vi "Blob Scoring.vi"(8 "HSL Image":T2, 11 "Acceptable Blobs":T4(array[cluster])) -> (3 "Acceptable Blobs + Scores":T3(array[cluster]))   [LabVIEW 2014]
uses:
  <vilib>/vision/Image Controls.llb/IMAQ Image.ctl
  <vilib>/vision/NI_Vision_Development_Module.lvlib
panel:
  in  "Particle Report":T1
  in  "Upper Limit Y":dbl[](array[numeric])
  in  "Lower Limit Y":dbl[](array[numeric])=[0.7, 0.7, 0.7, 0.7, 0.7, 0.7, 0.2, 0.2, 0.2, 0.2, 0.2, 0.2, 0.2, 0.2, 0.2, 0.2, 0.2, 0.2, 0.2, 0.2, 0.2]
  in  "Upper Limit X":dbl[](array[numeric])
  in  "Lower Limit X":dbl[](array[numeric])
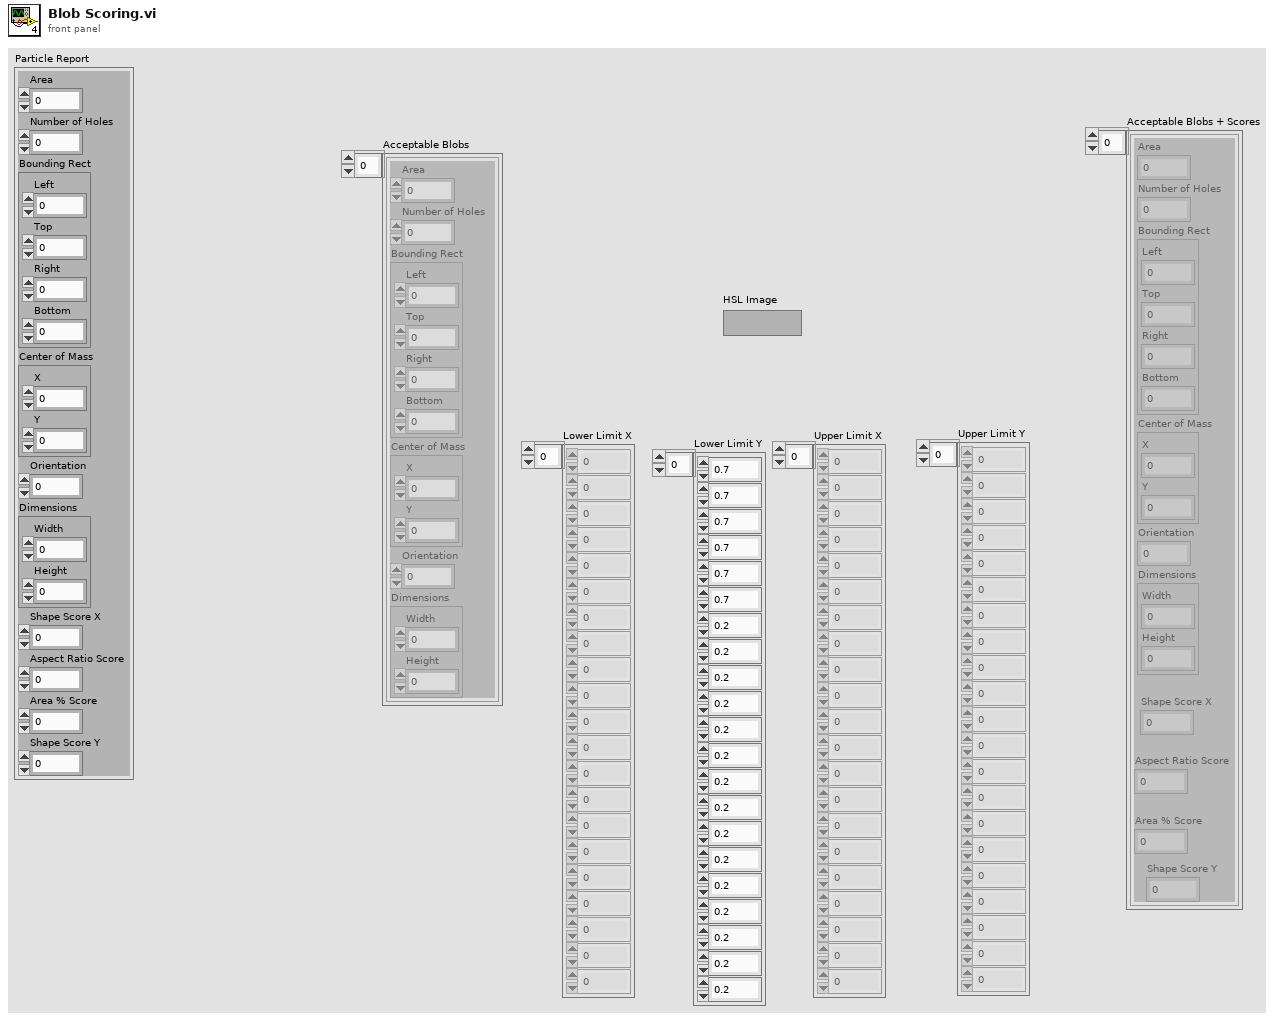
[diagram p1: front panel]
types:
  T1 = cluster{"Area":dbl, "Number of Holes":dbl, "Bounding Rect":cluster{"Left":dbl, "Top":dbl, "Right":dbl, "Bottom":dbl}, "Center of Mass":cluster{"X":dbl, "Y":dbl}, "Orientation":dbl, "Dimensions":cluster{"Width":dbl, "Height":dbl}, "Shape Score X":dbl, "Aspect Ratio Score":dbl, "Area % Score":dbl, "Shape Score Y":dbl}
  T2 = typedef "IMAQ Image.ctl" = refnum<image>
  T3 = cluster{"Area":dbl, "Number of Holes":dbl, "Bounding Rect":cluster{"Left":dbl, "Top":dbl, "Right":dbl, "Bottom":dbl}, "Center of Mass":cluster{"X":dbl, "Y":dbl}, "Orientation":dbl, "Dimensions":cluster{"Width":dbl, "Height":dbl}, "Shape Score X":dbl, "Aspect Ratio Score":dbl, "Area % Score":dbl, "Shape Score Y":dbl}[]
  T4 = cluster{"Area":dbl, "Number of Holes":dbl, "Bounding Rect":cluster{"Left":dbl, "Top":dbl, "Right":dbl, "Bottom":dbl}, "Center of Mass":cluster{"X":dbl, "Y":dbl}, "Orientation":dbl, "Dimensions":cluster{"Width":dbl, "Height":dbl}}[]
  T5 = cluster{"Left":dbl, "Top":dbl, "Right":dbl, "Bottom":dbl}
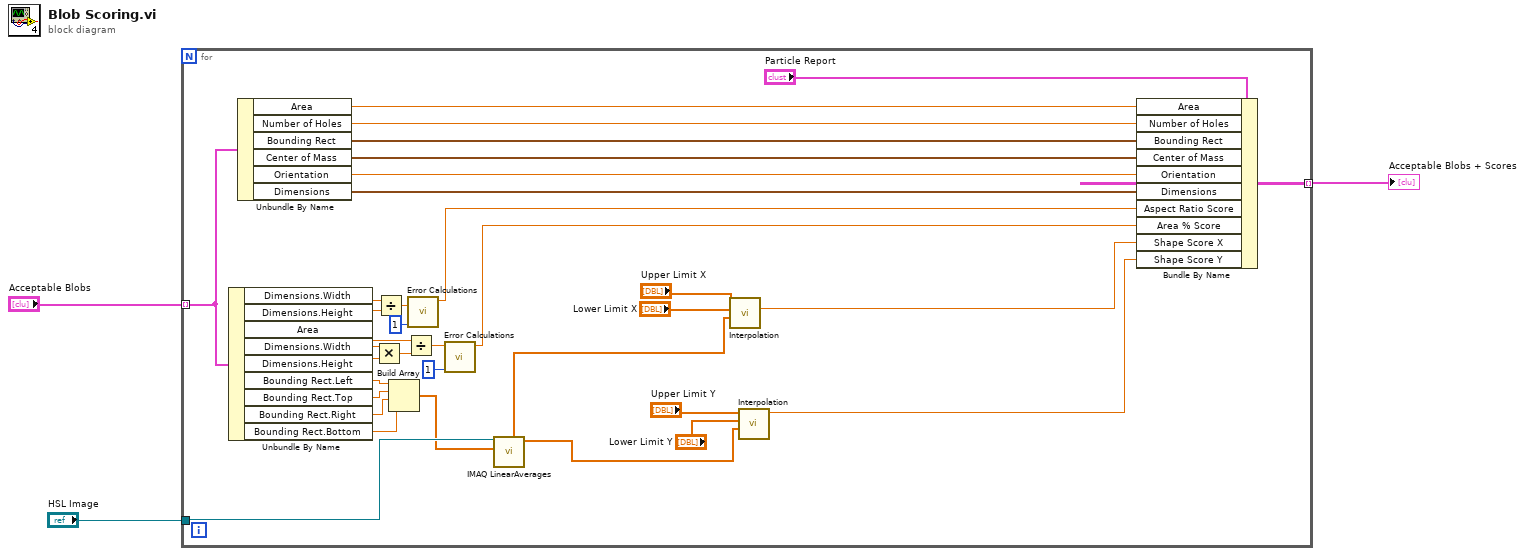
[diagram p0: block diagram]
diagram:
  n1 = for {
    tunnel: "Acceptable Blobs" -> [w21] mode=indexing
    tunnel: "HSL Image" -> [w28]
    tunnel: [w12] -> w1 mode=indexing
    n2 = Unbundle By Name(w21) -> ("Dimensions.Width"=w35:dbl, "Dimensions.Height"=w36:dbl, "Area"=w31:dbl, "Dimensions.Width"=w34:dbl, "Dimensions.Height"=w33:dbl, "Bounding Rect.Left"=w27:dbl, "Bounding Rect.Top"=w26:dbl, "Bounding Rect.Right"=w25:dbl, "Bounding Rect.Bottom"=w24:dbl)
    n3 = Unbundle By Name(w21) -> ("Area"=w20:dbl, "Number of Holes"=w19:dbl, "Bounding Rect"=w18:T5, "Center of Mass"=w17:cluster{"X":dbl, "Y":dbl}, "Orientation"=w16:dbl, "Dimensions"=w15:cluster{"Width":dbl, "Height":dbl})
    n4 = Multiply(x=w34, y=w33) -> (x*y=w32:dbl)
    n5 = Divide(x=w35, y=w36) -> (x/y=w37:dbl)
    n6 = Build Array(w27, w26, w25, w24) -> (w23:dbl[])
    n7 = Divide(x=w31, y=w32) -> (x/y=w30:dbl)
    n8 = call "Error Calculations.vi"("Accepted"=1, "Measured"=w37) -> ("Error"=w14:dbl)  [unwired: 9 in]
    n9 = call "Error Calculations.vi"("Accepted"=1, "Measured"=w30) -> ("Error"=w13:dbl)  [unwired: 9 in]
    n10 = call "IMAQ LinearAverages"("Optional Rectangle"=w23, "Image Src"=w28) -> ("Y Axis Averages"=w6:sgl[], "X Axis Averages"=w9:sgl[])  [unwired: 5 in, 3 out]
    n11 = call "Interpolation.vi"("Real Data"=w9, "Lower Limit"="Lower Limit X", "Upper Limit"="Upper Limit X") -> ("instances of true"=w4:dbl)  [unwired: 8 in]
    n12 = call "Interpolation.vi"("Real Data"=w6, "Lower Limit"="Lower Limit Y", "Upper Limit"="Upper Limit Y") -> ("instances of true"=w5:dbl)  [unwired: 8 in]
    n13 = Bundle By Name(cluster="Particle Report", "Area"=w20, "Number of Holes"=w19, "Bounding Rect"=w18, "Center of Mass"=w17, "Orientation"=w16, "Dimensions"=w15, "Aspect Ratio Score"=w14, "Area % Score"=w13, "Shape Score X"=w4, "Shape Score Y"=w5) -> (w12:T1)
  }
  "Acceptable Blobs + Scores" <- w1
